vi "End Sound.vi"   [LabVIEW 2021]
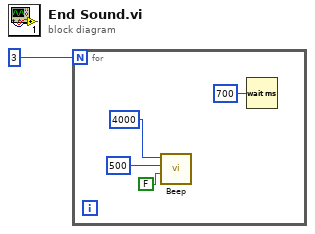
[diagram p0: block diagram]
diagram:
  n1 = for {
    N: 3 -> [_]
    n2 = call <vilib>:"Beep.vi"("use system alert? (T)"=FALSE, "duration (msec)"=u32 500, "frequency (Hz)"=u32 4000) -> ()  [unwired: 9 in]
    n3 = Wait (ms)(milliseconds to wait=u32 700) -> ()  [unwired: 1 out]
  }
